vi "STARTREADY.vi"() -> ()   [LabVIEW 2024]
uses:
  <vilib>/Utility/file.llb/Read Delimited Spreadsheet (DBL).vi
panel:
  in  "Flow Rate Lower Limit 2":dbl
  in  "Flow Rate Upper Limit 2":dbl
  in  "Desired Flow Rate 3":dbl format="%_2f"
  in  "Initial RPM  3":dbl format="%_4f"
  in  "stop 2":bool
  out "Boolean":bool
  out "Waveform Chart 3":dbl[](graph)
  out "Waveform Chart 2":dbl[](graph)
  out "Flow Rate":dbl[](graph)
  in  "Color Box":u32(colorbox)
  # "Blood Flow Rate"
  # "Flow Rate (mL/min)"
  # "Initial LVAD Speed (RPM)"
  # "Desired Flow Rate (mL/min)"
  # "LVAD Speed"
  # "Upper Flow Rate Limit (mL/min)"
  # "Speed (RPM)"
  # "Lower Flow Rate Limit (mL/min)"
  # "Optimal Flow State"
  # "Right Heart Waveform"
  # "Amplitude"
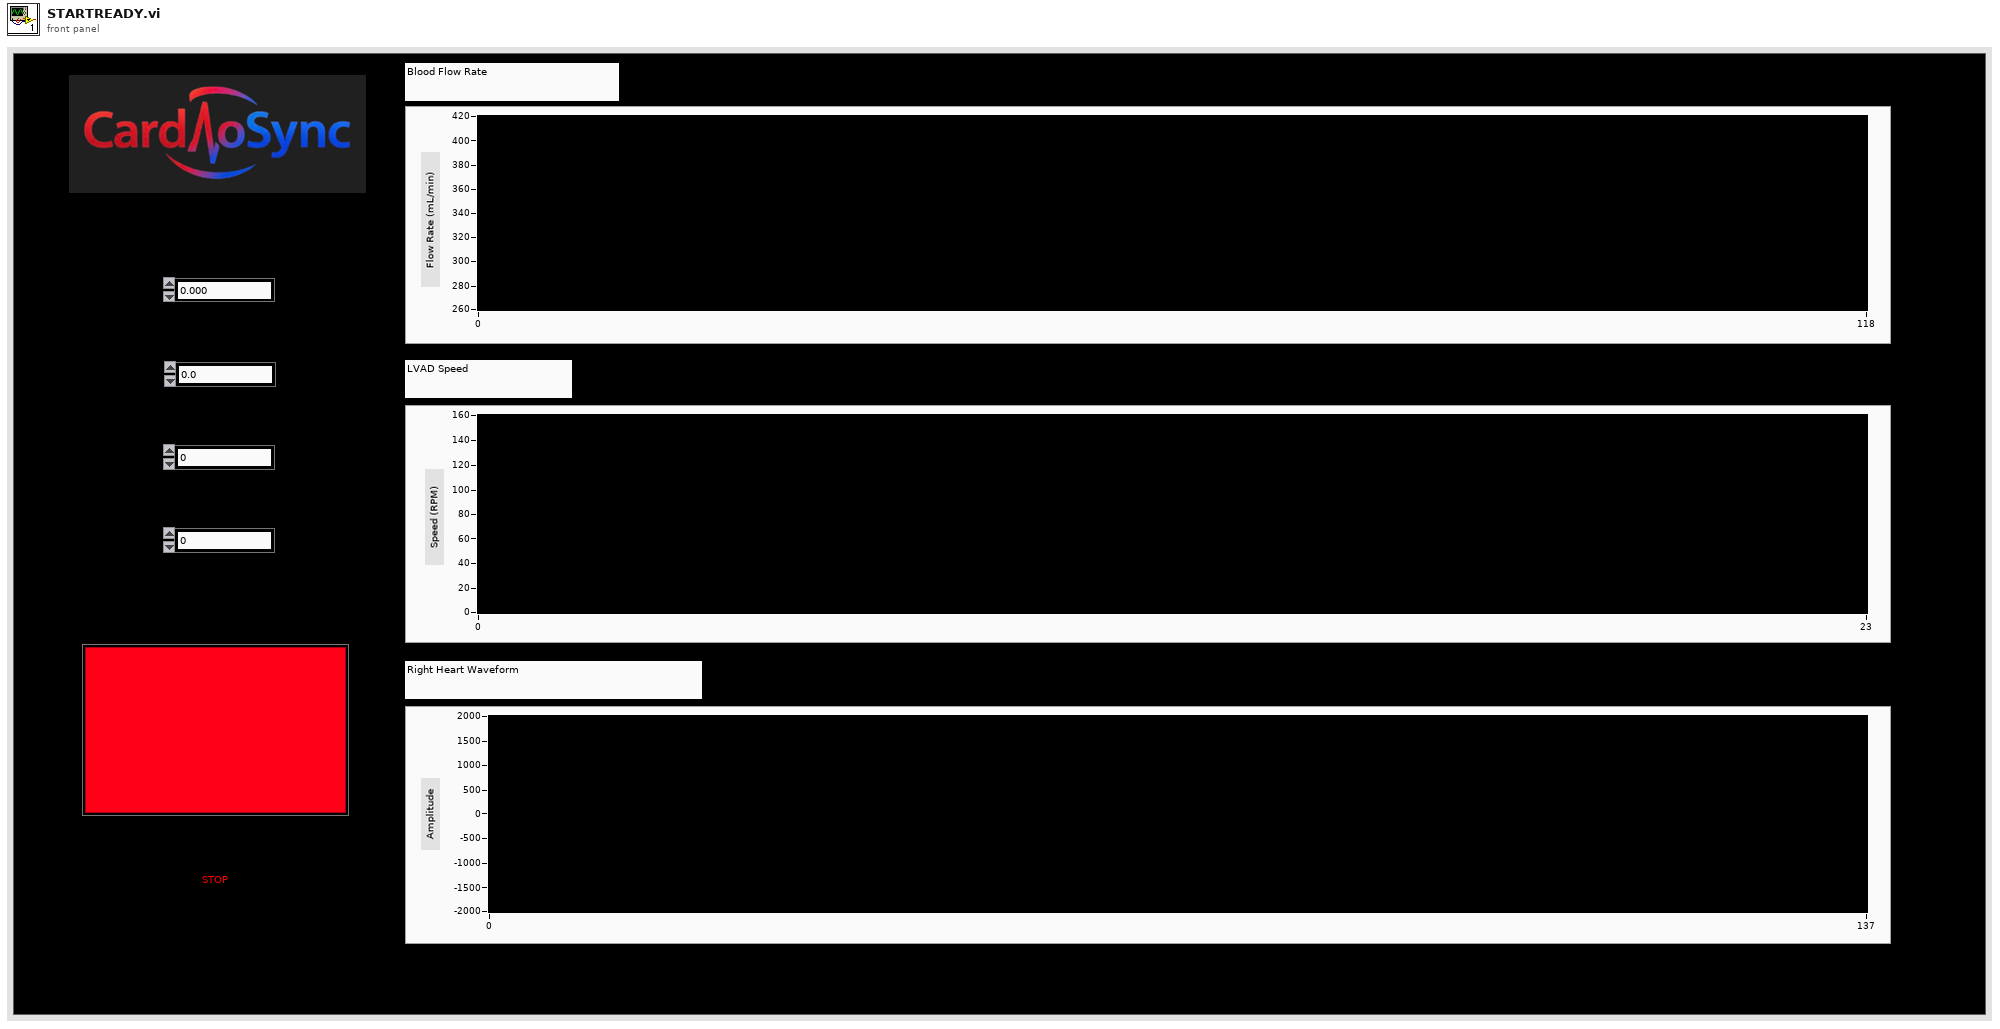
[diagram p1: front panel]
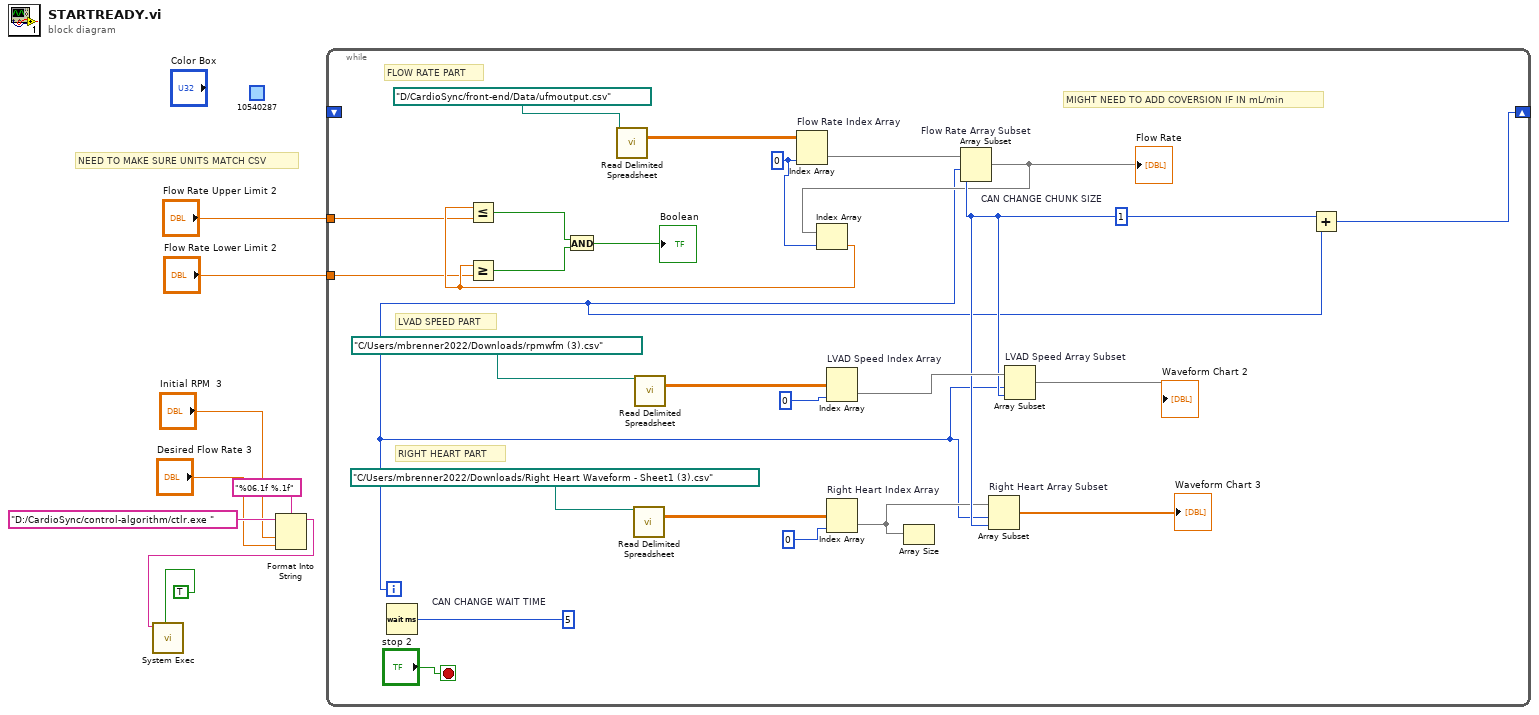
[diagram p0: block diagram]
diagram:
  (unwired) u32 10540287 ("Color Box 2")
  # "NEED TO MAKE SURE UNITS MATCH CSV"
  n1 = Format Into String(format string="%06.1f %.1f", initial string="D:/CardioSync/control-algorithm/ctlr.exe ", "Initial RPM  3", "Desired Flow Rate 3") -> (resulting string=w2:string)  [unwired: 1 in, 1 out]
  n2 = call <vilib>:"System Exec.vi"("wait until completion? (T)"=TRUE, "command line"=w2) -> ()  [unwired: 6 in, 4 out]
  n3 = while {
    shift-right: [w30] -> _
    shift-left: _ -> [_]
    tunnel: "Flow Rate Upper Limit 2" -> [w11]
    tunnel: "Flow Rate Lower Limit 2" -> [w10]
    i -> [w9]
    stop <- "stop 2" stop-if-true
    w31 = u32 5  # CAN CHANGE WAIT TIME
    w23 = 1  # CAN CHANGE CHUNK SIZE
    w14 = 0 ("disabled index (col)")
    # "MIGHT NEED TO ADD COVERSION IF IN mL/min"
    # "RIGHT HEART PART"
    # "LVAD SPEED PART"
    # "FLOW RATE PART"
    n4 = Wait (ms)(milliseconds to wait=w31) -> ()  [unwired: 1 out]
    n5 = call-poly <vilib>:"Read Delimited Spreadsheet.vi"("file path (dialog if empty)"=path "D:/CardioSync/front-end/Data/ufmoutput.csv") -> ("all rows"=w33:dbl[][])  [unwired: 9 in, 5 out]
    n6 = call-poly <vilib>:"Read Delimited Spreadsheet.vi"("file path (dialog if empty)"=path "C:/Users/mbrenner2022/Downloads/Right Heart Waveform - Sheet1 (3).csv") -> ("all rows"=w24:dbl[][])  [unwired: 9 in, 5 out]
    n7 = call-poly <vilib>:"Read Delimited Spreadsheet.vi"("file path (dialog if empty)"=path "C:/Users/mbrenner2022/Downloads/rpmwfm (3).csv") -> ("all rows"=w27:dbl[][])  [unwired: 9 in, 5 out]
    n8 = Index Array "Flow Rate Index Array"(array=w33, index (col)=w14) -> (element=w32:dbl[])  [unwired: 1 in]
    n9 = Index Array "LVAD Speed Index Array"(array=w27, index (col)=0 ("disabled index (col)")) -> (element=w26:dbl[])  [unwired: 1 in]
    n10 = Index Array "Right Heart Index Array"(array=w24, index (col)=0 ("disabled index (col)")) -> (element=w19:dbl[])  [unwired: 1 in]
    n11 = Array Size(array=w19) -> ()  [unwired: 1 out]
    n12 = Array Subset "Flow Rate Array Subset"(array=w32, index=w9, length=w23) -> (w15:dbl[])
    "Flow Rate" <- w15
    n13 = Index Array(array=w15, index=w14) -> (element=w13:dbl)
    n14 = Less Or Equal?(x=w13, y=w11) -> (x <= y?=w18:bool)
    n15 = Greater Or Equal?(x=w13, y=w10) -> (x >= y?=w17:bool)
    n16 = And(x=w18, y=w17) -> (x .and. y?=→"Boolean":bool)
    n17 = Array Subset "Right Heart Array Subset"(array=w19, index=w9, length=w23) -> (→"Waveform Chart 3":dbl[])
    n18 = Array Subset "LVAD Speed Array Subset"(array=w26, index=w9, length=w23) -> (→"Waveform Chart 2":dbl[])
    n19 = Add(x=w23, y=w9) -> (x+y=w30:i32)
  }
